vi "Read Current Status Msg.vi"(11 "EMS Generic":refnum<class "EMS Generic.lvclass">) -> (2 "Return Current Status Msg":refnum<class "Return String Msg.lvclass">, 3 "dup EMS Generic":refnum<class "EMS Generic.lvclass">)   [LabVIEW 2018, in "EMS Generic Actor.lvlib" / "EMS Generic.lvclass"]
uses:
  EMS Generic.lvclass
  EMS Generic Messages/Return String Msg/Return String Msg.lvclass
  EMS Generic.lvclass/EMS Generic.ctl
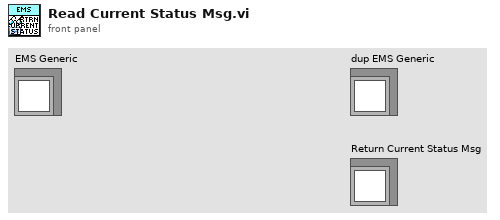
[diagram p1: front panel]
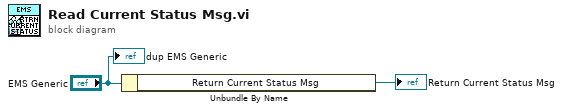
[diagram p0: block diagram]
diagram:
  n1 = Unbundle By Name("EMS Generic") -> ("Return Current Status Msg"=→"Return Current Status Msg":refnum<class "Return String Msg.lvclass">)
  "dup EMS Generic" <- "EMS Generic"
